vi "Parse CfgTable.vi"(7 "Cluster Configuration Typedef":variant, 8 "error in (no error)":errorcluster, 11 "CfgTable Row":string[](array[string])) -> (0 "error out":errorcluster, 3 "Cluster Configuration Out":variant)   [LabVIEW 2017, in "ClusterCfgTable.lvlib"]
uses:
  ClusterCfgTable.lvlib
  <userlib>/_OpenG.lib/string/string.llb/Trim Whitespace (String)__ogtk.vi
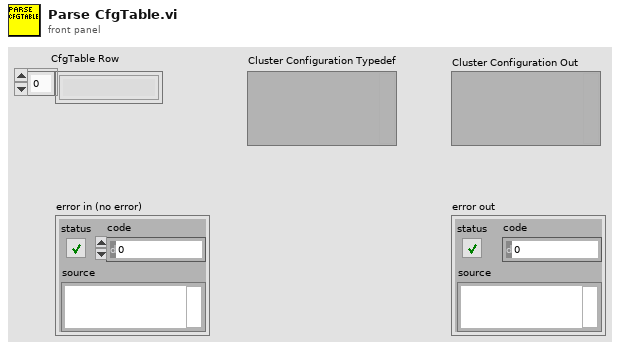
[diagram p1: front panel]
types:
  T1 = typedef "Type Descriptor Enumeration__ogtk.ctl" = enum8{"<Null>", "I8", "I16", "I32", "I64", "U8", "U16", "U32", "U64", "SGL", "DBL", "EXT", "CSG", "CDB", "CXT", "0x0F", "0x10", "0x11", "0x12", "0x13", "0x14", "Enum U8", "Enum U16", "Enum U32", "Enum U64", "SGL PQ", "DBL PQ", "EXT PQ", "CSG PQ", "CDB PQ", "CXT PQ", "0x1F", "0x20", "Boolean", "0x22", "0x23", "0x24", "0x25", "0x26", "0x27", "0x28", "0x29", "0x2A", "0x2B", "0x2C", "0x2D", "0x2E", "0x2F", "String", "0x31", "Path", "Pict", "0x34", "0x35", "0x36", "DAQ", "0x38", "0x39", "0x3A", "0x3B", "0x3C", "0x3D", "0x3E", "0x3F", "Array", "0x41", "0x42", "0x43", "0x44", "0x45", "0x46", "0x47", "0x48", "0x49", "0x4A", "0x4B", "0x4C", "0x4D", "0x4E", "0x4F", "Cluster", "0x51", "0x52", "Variant", "Waveform", "0x55", "0x56", "0x57", "0x58", "0x59", "0x5A", "0x5B", "0x5C", "0x5D", "0x5E", "0x5F", "0x60", "0x61", "0x62", "0x63", "0x64", "0x65", "0x66", "0x67", "0x68", "0x69", "0x6A", "0x6B", "0x6C", "0x6D", "0x6E", "0x6F", "Refnum"}
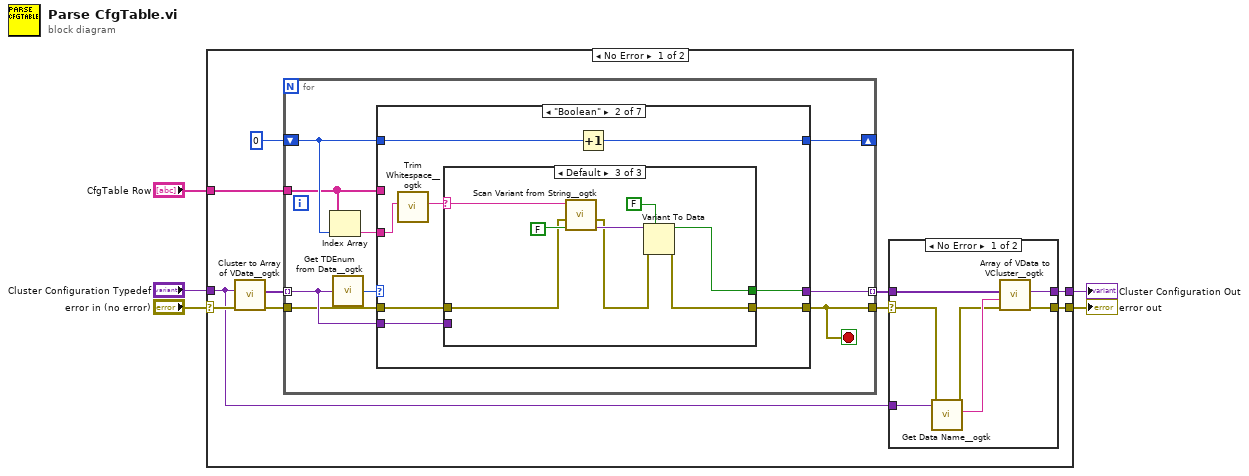
[diagram p0: block diagram]
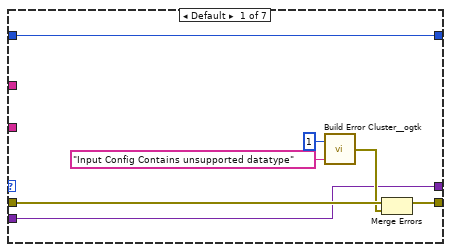
[diagram p3: hidden frame]
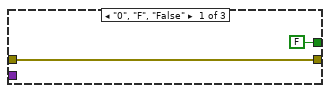
[diagram p4: hidden frame]
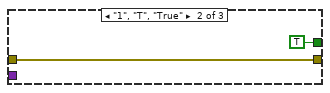
[diagram p5: hidden frame]
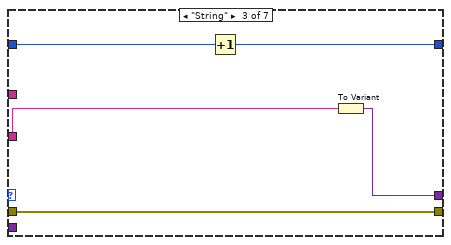
[diagram p6: hidden frame]
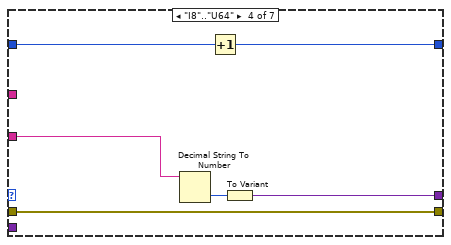
[diagram p7: hidden frame]
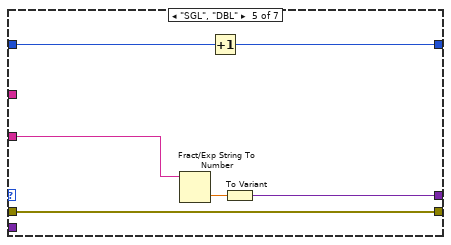
[diagram p8: hidden frame]
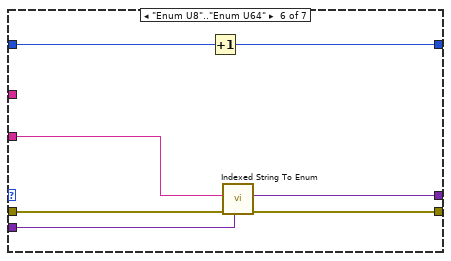
[diagram p9: hidden frame]
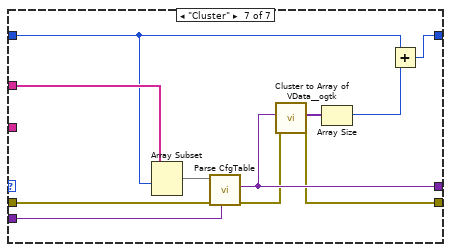
[diagram p10: hidden frame]
diagram:
  n1 = case shown="No Error" "error in (no error)" {
    selector: "error in (no error)" -> [w10 w97]
    tunnel: "CfgTable Row" -> [w15 _]
    tunnel: [w14 w96] -> w4
    tunnel: [w13 w97] -> w3
    tunnel: "Cluster Configuration Typedef" -> [w6 w96]
    frame No Error {
      n2 = call <userlib>:"Cluster to Array of VData__ogtk.vi"("error in (no error)"=w10, "Cluster"=w6) -> ("error out"=w11:errorcluster, "Array of VData"=w8:variant[])  [unwired: 8 in]
      n3 = for {
        tunnel: w15 -> [w25]
        tunnel: w8 -> [w30] mode=indexing
        tunnel: [w31] -> w9 mode=indexing
        tunnel: w11 -> [w29]
        tunnel: [w28] -> w12
        shift-right: [w27] -> _
        shift-left: 0 -> [w26]
        stop <- w28 stop-if-true
        n4 = Index Array(array=w25, index=w26) -> (element=w32:string)
        n5 = call <userlib>:"Get TDEnum from Data__ogtk.vi"("Data"=w30) -> ("Type Descriptor Enumeration"=w33:T1)  [unwired: 4 in]
        n6 = case shown="\"Boolean\"" w33 {
          tunnel: w32 -> [_ w48 w65 w70 w76 w84 _]
          tunnel: [w35 w46 w64 w71 w77 w83 w90] -> w31
          tunnel: w30 -> [w35 w47 _ _ _ w82 w92]
          tunnel: w29 -> [w40 w44 w63 w68 w74 w81 w95]
          tunnel: [w39 w43 w63 w68 w74 w80 w85] -> w28
          tunnel: w26 -> [w34 w42 w62 w67 w73 w79 w88]
          tunnel: [w34 w41 w61 w66 w72 w78 w87] -> w27
          tunnel: w25 -> [_ _ _ _ _ _ w94]
          frame Default {
            n7 = call <userlib>:"Build Error Cluster__ogtk.vi"("String to Prepend to source (\"\")"="Input Config Contains unsupported datatype" ("String to Prepend to source (\"\")"), "code"=1) -> ("error out"=w38:errorcluster)
            n8 = Merge Errors(w40, w38) -> (w39:errorcluster)
          }
          frame "Boolean" {
            n9 = call-poly <userlib>:"Trim Whitespace__ogtk.vi"("String in"=w48) -> ("String out"=w45:string)  [unwired: 6 in]
            n10 = case shown="Default" w45 {
              selector: w45 -> [_ _ w60]
              tunnel: w47 -> [_ _ _]
              tunnel: [FALSE TRUE w57] -> w46
              tunnel: w44 -> [w49 w51 w55]
              tunnel: [w49 w51 w53] -> w43
              frame "0", "F", "False" {
              }
              frame "1", "T", "True" {
              }
              frame Default {
                n11 = call <userlib>:"Scan Variant from String__ogtk.vi"("Default Value"=FALSE, "error in (no error)"=w55, "Input String"=w60) -> ("Output"=w59:variant, "error out"=w54:errorcluster)  [unwired: 5 in, 2 out]
                n12 = Variant To Data(error in=w54, type=FALSE, Variant=w59) -> (data=w57:bool, error out=w53:errorcluster)
              }
            }
            n13 = Increment(x=w42) -> (x+1=w41:i32)
          }
          frame "String" {
            n14 = Increment(x=w62) -> (x+1=w61:i32)
            n15 = To Variant(anything=w65) -> (Variant=w64:variant)
          }
          frame "I8".."U64" {
            n16 = Decimal String To Number(string=w70) -> (number=w69:i32)  [unwired: 2 in, 1 out]
            n17 = Increment(x=w67) -> (x+1=w66:i32)
            n18 = To Variant(anything=w69) -> (Variant=w71:variant)
          }
          frame "SGL", "DBL" {
            n19 = Fract/Exp String To Number(string=w76) -> (number=w75:dbl)  [unwired: 3 in, 1 out]
            n20 = Increment(x=w73) -> (x+1=w72:i32)
            n21 = To Variant(anything=w75) -> (Variant=w77:variant)
          }
          frame "Enum U8".."Enum U64" {
            n22 = Increment(x=w79) -> (x+1=w78:i32)
            n23 = call "Indexed String To Enum.vi"("Variant"=w82, "error in (no error)"=w81, "String"=w84) -> ("error out"=w80:errorcluster, "Enum"=w83:variant)  [unwired: 7 in]
          }
          frame "Cluster" {
            n24 = Array Subset(array=w94, index=w88) -> (w93:string[])  [unwired: 1 in]
            n25 = call "Parse CfgTable.vi"("Cluster Configuration Typedef"=w92, "error in (no error)"=w95, "CfgTable Row"=w93) -> ("error out"=w86:errorcluster, "Cluster Configuration Out"=w90:variant)  [unwired: 7 in]
            n26 = call <userlib>:"Cluster to Array of VData__ogtk.vi"("error in (no error)"=w86, "Cluster"=w90) -> ("error out"=w85:errorcluster, "Array of VData"=w91:variant[])  [unwired: 8 in]
            n27 = Array Size(array=w91) -> (size(s)=w89:i32)
            n28 = Add(x=w88, y=w89) -> (x+y=w87:i32)
          }
        }
      }
      n29 = case shown="No Error" w12 {
        selector: w12 -> [w17 w23]
        tunnel: [w22 w24] -> w14
        tunnel: [w21 w23] -> w13
        tunnel: w9 -> [w20 _]
        tunnel: w6 -> [w18 w24]
        frame No Error {
          n30 = call <userlib>:"Get Data Name__ogtk.vi"("error in (no error)"=w17, "Data"=w18) -> ("error out"=w16:errorcluster, "Data Name"=w19:string)  [unwired: 7 in, 1 out]
          n31 = call <userlib>:"Array of VData to VCluster__ogtk.vi"("error in (no error)"=w16, "Cluster Name"=w19, "Array"=w20) -> ("error out"=w21:errorcluster, "VCluster"=w22:variant)  [unwired: 7 in]
        }
        frame Error {
        }
      }
    }
    frame Error {
    }
  }
  "Cluster Configuration Out" <- w4
  "error out" <- w3
